vi "Real-Time LED-Core_Process.vi"(0 "FTW Actor Instance Configuration":string="{\n  \"Identity\": \"RT LED\",\n  \"InboxAddress\": \"inproc://rt-led\",\n  \"LoggerAddress\": \"\"\n}", 11 "ErrorIn":errorcluster) -> (15 "Error":errorcluster)   [LabVIEW 2015, in "Real-Time LED-Core.lvclass"]
uses:
  Real-Time LED-Core.lvclass
  Real-Time LED-Core.lvclass/Real-Time LED-Core.ctl
  source/actor/Instance/FTW-ActorInstance.lvclass/FTW-ActorInstance.ctl
  source/actor/JobSequencer/FTW-SEQ-Current.vi
  source/actor/Instance/FTW-ActorInstance.lvclass
  source/actor/Message/Request/FTW-Message-IncomingRequest.lvclass
  <vilib>/NI_Real-Time Target Support.lvlib
panel:
  out "LED":bool
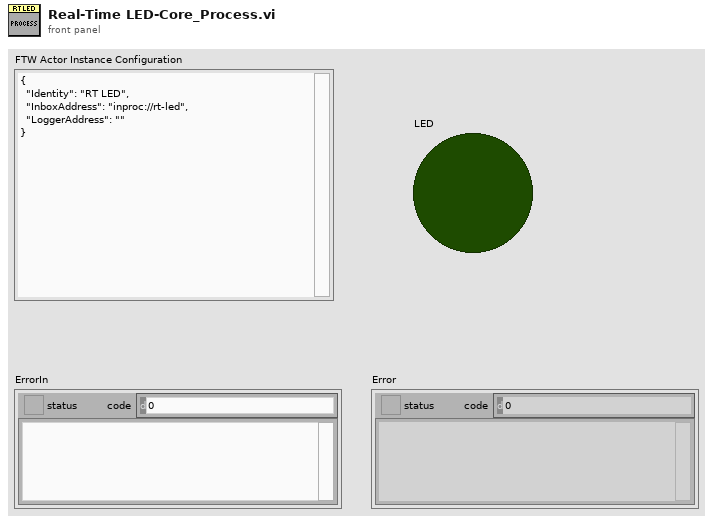
[diagram p1: front panel]
types:
  T1 = cluster{"Incoming Requests":refnum<event-registration>, "Local Messages":refnum<event-registration>, "Subscriber Registration":refnum<event-registration>}
  T2 = cluster{"Period":i32, "Sequence":bool[], "Color":i32}
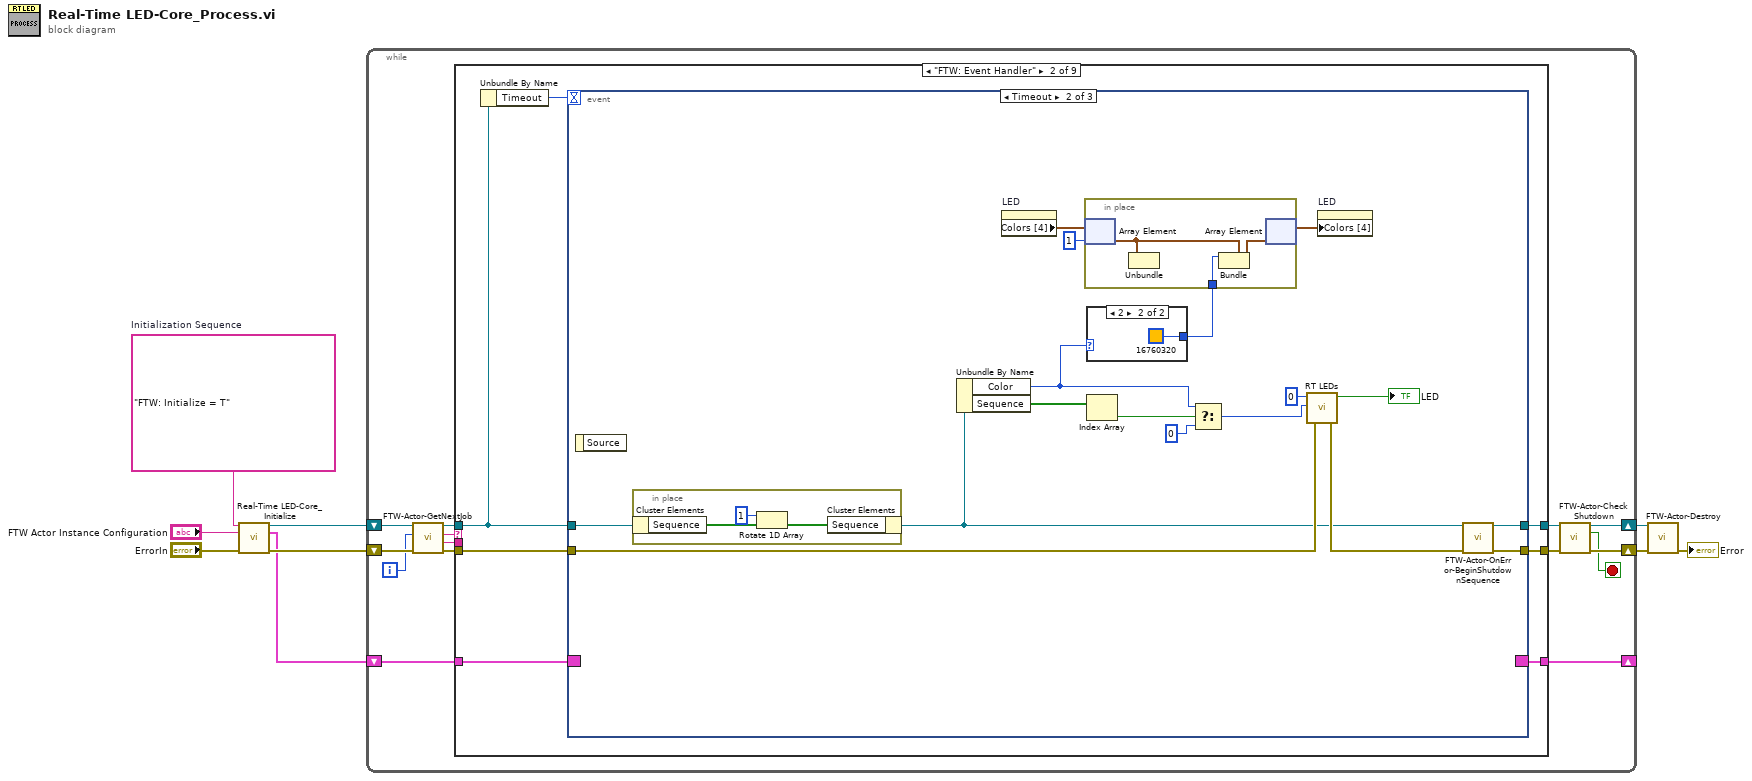
[diagram p0: block diagram]
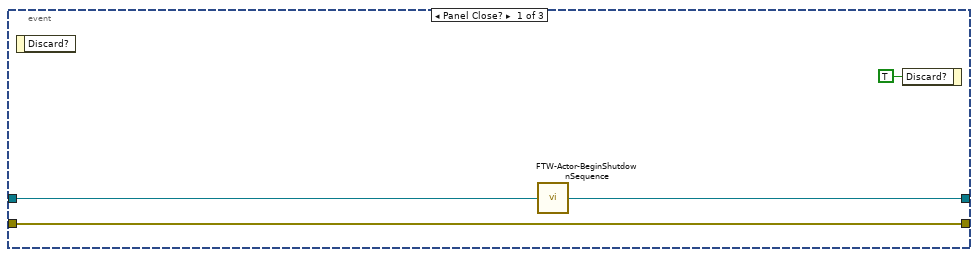
[diagram p3: hidden frame]
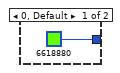
[diagram p4: hidden frame]
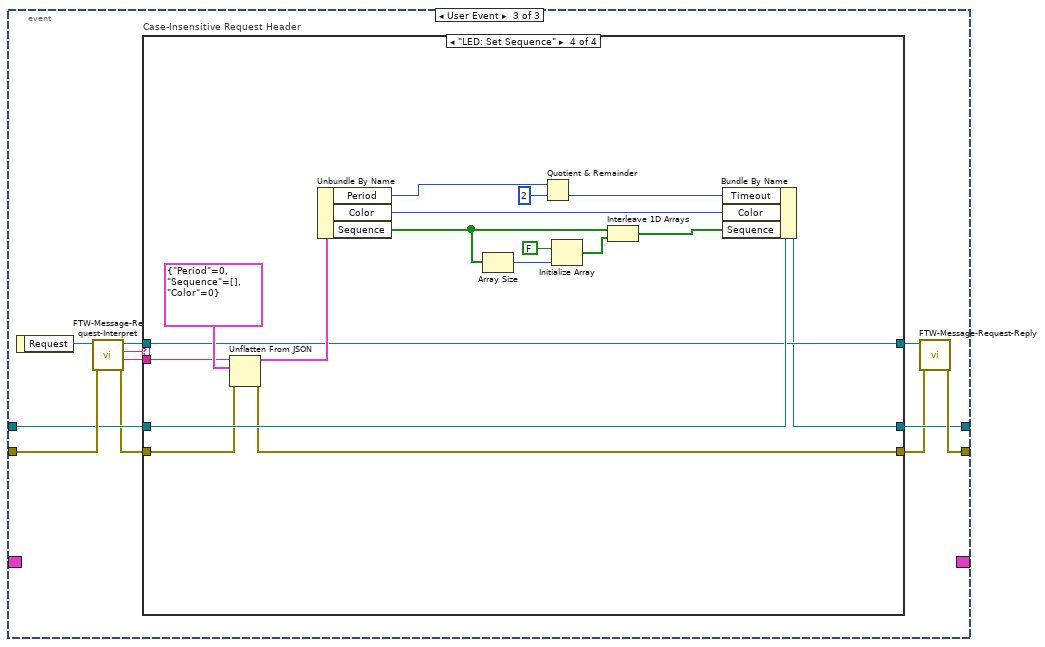
[diagram p5: hidden frame]
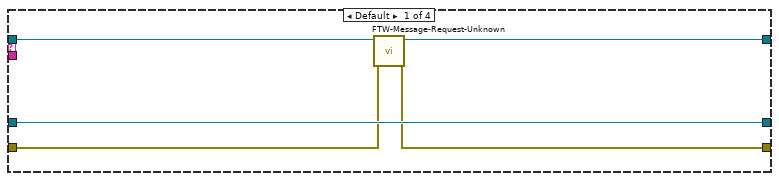
[diagram p6: hidden frame]
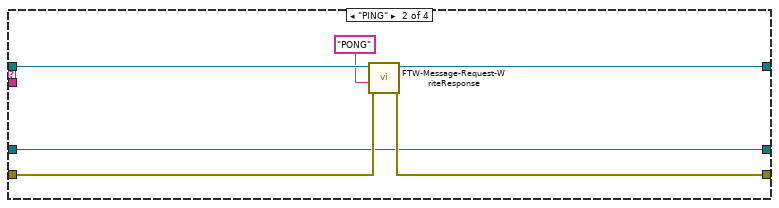
[diagram p7: hidden frame]
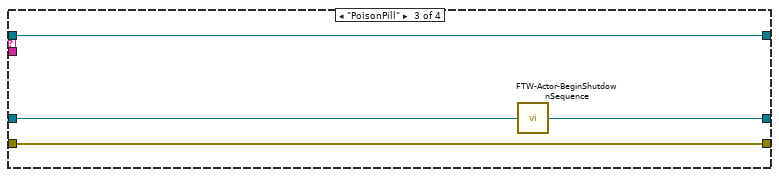
[diagram p8: hidden frame]
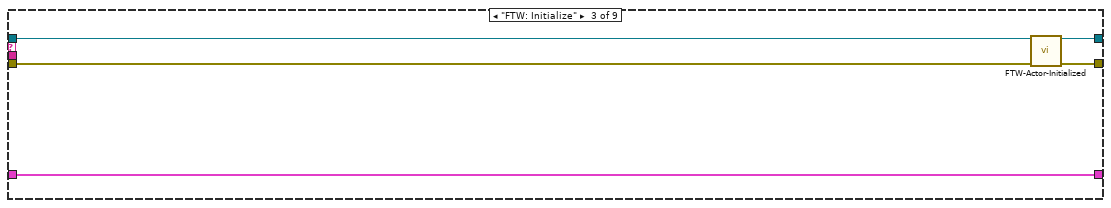
[diagram p9: hidden frame]
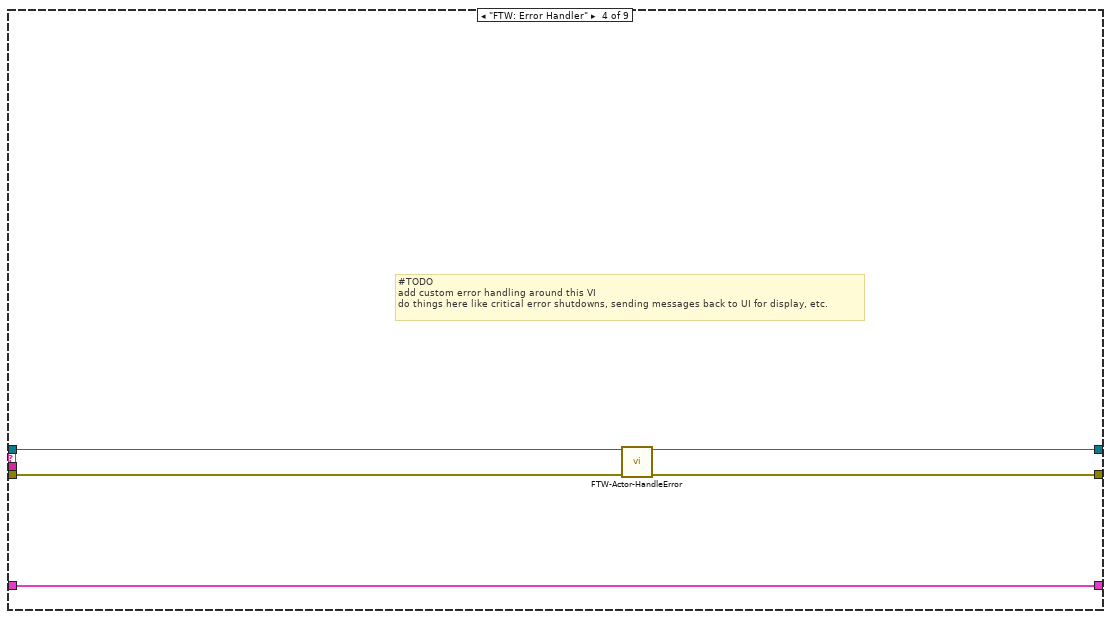
[diagram p10: hidden frame]
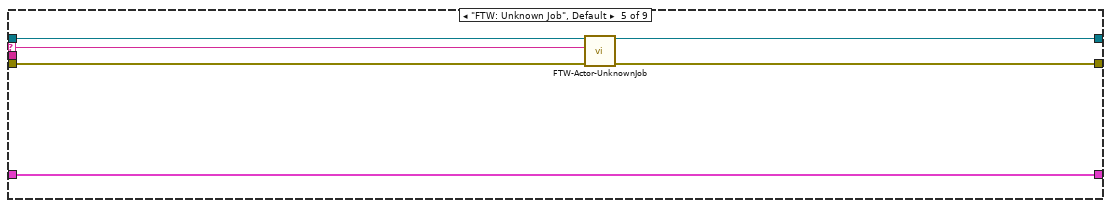
[diagram p11: hidden frame]
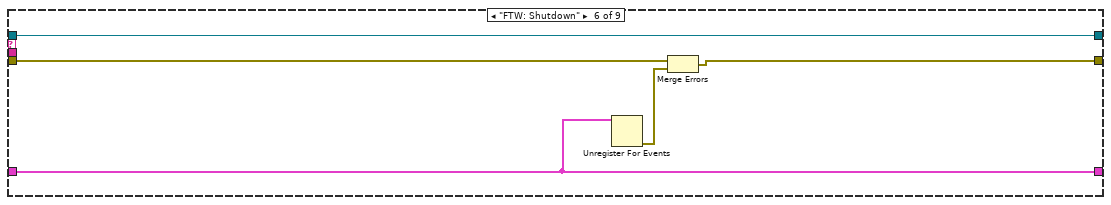
[diagram p12: hidden frame]
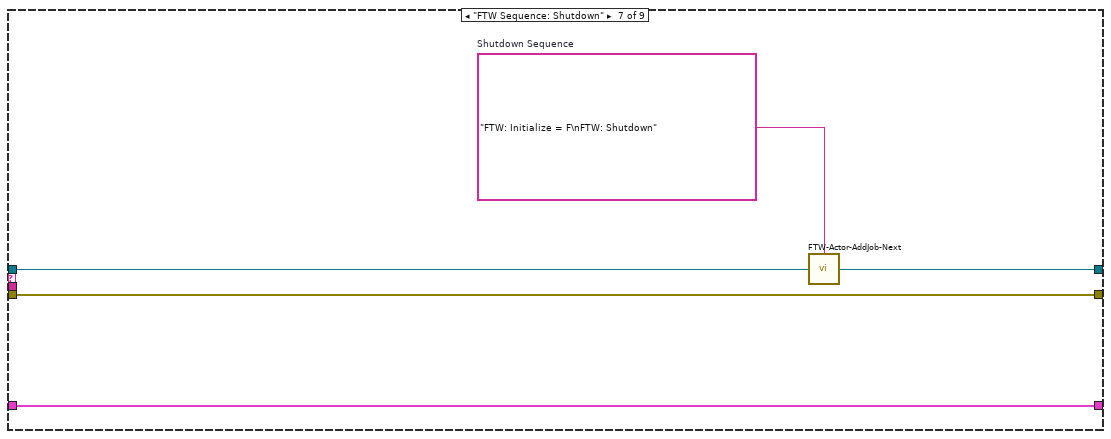
[diagram p13: hidden frame]
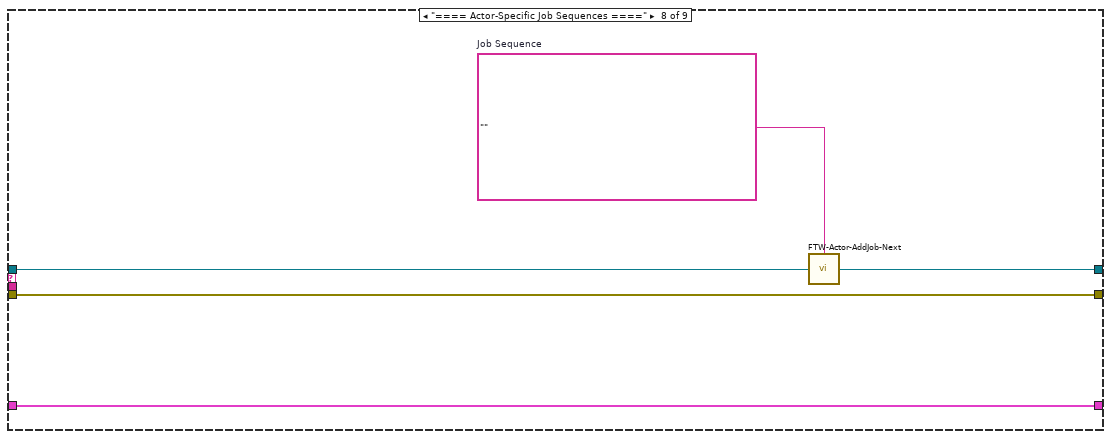
[diagram p14: hidden frame]
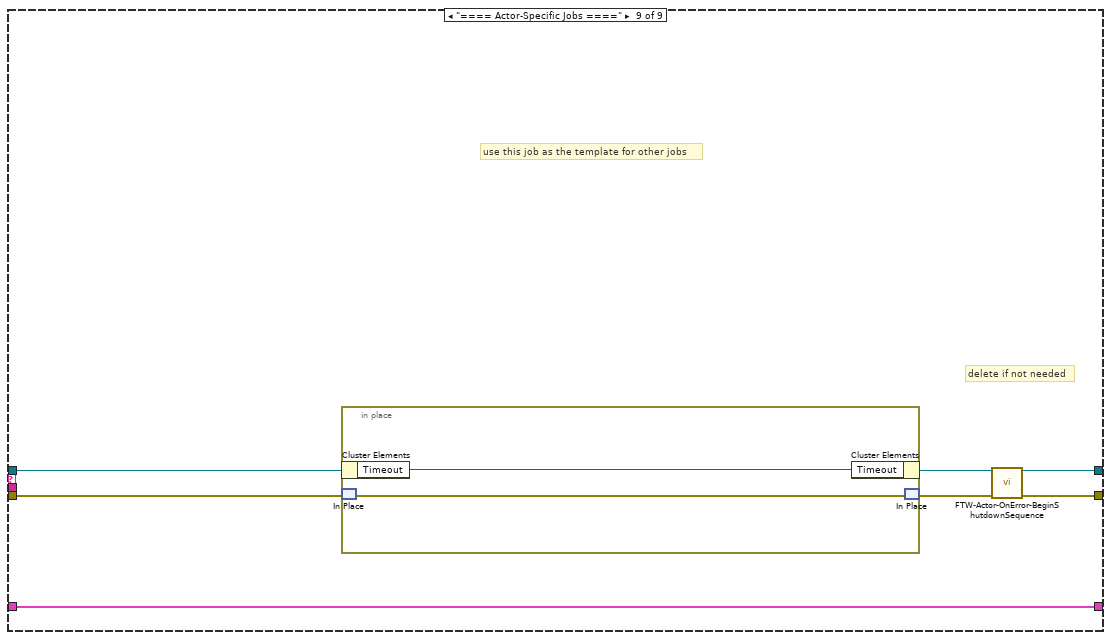
[diagram p15: hidden frame]
diagram:
  w5 = "FTW: Initialize = T"  # Initialization Sequence
  n1 = call "Real-Time LED-Core_Initialize.vi"("Initialization Sequence"=w5, "FTW Actor Instance Configuration"="FTW Actor Instance Configuration", "error in (no error)"="ErrorIn") -> ("Actor Template-Core out"=w1:refnum<class "Real-Time LED-Core.lvclass">, "Event Refnums"=w2:T1, "error out"=w6:errorcluster)  [unwired: 10 in]
  n2 = while {
    shift-right: [w13] -> w8
    shift-left: w6 -> [w20]
    shift-right: [w10] -> _
    shift-left: w2 -> [w23]
    shift-right: [w15] -> w9
    shift-left: w1 -> [w22]
    i -> [w11]
    stop <- w12 stop-if-true
    n3 = call "FTW-Actor-GetNextJob.vi"("error in"=w20, "Jobs Performed"=w11, "FTW Actor Instance"=w22) -> ("error out"=w19:errorcluster, "Job Data"=w17:string, "Job Name"=w18:string, "FTW Actor Instance out"=w21:refnum<class "Real-Time LED-Core.lvclass">)  [unwired: 5 in]
    n4 = case shown="\"FTW: Event Handler\"" w18 {
      selector: w18 -> [_ _ _ _ w116 _ _ _ _]
      tunnel: [w25 w33 w107 w111 w119 w125 w130 w135 w139] -> w14
      tunnel: w19 -> [w25 w32 w109 w113 w120 w126 w130 w135 w142]
      tunnel: w23 -> [w26 w29 w110 w115 w121 w123 w131 w136 w143]
      tunnel: [w26 w31 w110 w115 w121 w123 w131 w136 w143] -> w10
      tunnel: w17 -> [_ _ _ _ _ _ _ _ _]
      tunnel: [w24 w30 w108 w112 w117 w122 w128 w133 w137] -> w16
      tunnel: w21 -> [w24 w28 w106 w114 w118 w122 w129 w134 w140]
      frame "==== Featherweight Framework Jobs ====" {
      }
      frame "FTW: Event Handler" {
        n5 = Unbundle By Name(w28) -> ("Timeout"=w27:i32)
        n6 = event shown="[1] Timeout" {
          selector: w29 -> [_ _ _]
          dyn-events: [_ _ _] -> w31
          timeout: w27 -> [_ _ _]
          tunnel: [w36 w40 w72] -> w33
          tunnel: w32 -> [w36 w54 w71]
          tunnel: [w34 w39 w66] -> w30
          tunnel: w28 -> [w35 w50 w70]
          event Panel Close? {
            n7 = event-data() -> ()  [unwired: 1 in, 1 out]
            n8 = call "FTW-Actor-BeginShutdownSequence.vi"("FTW Actor Instance"=w35) -> ("FTW Actor Instance out"=w34:refnum<class "Real-Time LED-Core.lvclass">)  [unwired: 3 in]
            n9 = event-data("Discard?"=TRUE) -> ()  [unwired: 1 in, 1 out]
          }
          event Timeout {
            n10 = event-data() -> ()  [unwired: 1 in, 1 out]
            n11 = in-place {
              n12 = in-place-cluster #1(w50) -> ("Sequence"=w62:bool[])
              n13 = Rotate 1D Array(1:w62, 2:1 ("n")) -> (0:w61:bool[])
              n14 = in-place-cluster #1("Sequence"=w61) -> (w38:refnum<class "Real-Time LED-Core.lvclass">)
            }
            n15 = Unbundle By Name(w38) -> ("Color"=w43:i32, "Sequence"=w49:bool[])
            n16 = property on="LED" class="Bool (strict)"() -> ("Colors [4]"=w46:cluster{u32, u32}[])  [unwired: 2 in, 2 out]
            n17 = case shown="2" w43 {
              tunnel: [u32 6618880 u32 16760320] -> w42
              frame 0, Default {
              }
              frame 2 {
              }
            }
            n18 = in-place {
              in-place-border: w42 -> [w57]
              n19 = in-place-array #2(w46, 1) -> (w59:cluster{u32, u32})
              n20 = Unbundle(w59) -> ()  [unwired: 2 out]
              n21 = Bundle(cluster=w59, w57) -> (w58:cluster{u32, u32})  [unwired: 1 in]
              n22 = in-place-array #2(w58) -> (w44:cluster{u32, u32}[])  [unwired: 1 out]
            }
            n23 = Index Array(array=w49) -> (element=w48:bool)  [unwired: 1 in]
            n24 = Select(t=w43, s=w48, f=0) -> (s? t:f=w52:i32)
            n25 = call <vilib>:"RT LEDs.vi"("error in (no error)"=w54, "State"=w52, "LED Num"=0) -> ("error out"=w53:errorcluster, "Led State"=→"LED":bool)  [unwired: 3 in]
            n26 = property on="LED" class="Bool (strict)"("Colors [4]"=w44) -> ()  [unwired: 2 in, 2 out]
            n27 = call-dynamic "FTW-Actor-OnError-BeginShutdownSequence.vi"("FTW Actor Instance"=w38, "error in"=w53) -> ("FTW Actor Instance out"=w39:refnum<class "Real-Time LED-Core.lvclass">, "error out"=w40:errorcluster)  [unwired: 12 in]
          }
          event User Event {
            n28 = event-data() -> ("Request"=w73:refnum<class "FTW-Message-IncomingRequest.lvclass">)  [unwired: 1 in]
            n29 = call "FTW-Message-Request-Interpret.vi"("error in"=w71, "FTW Incoming Request"=w73) -> ("error out"=w69:errorcluster, "Request Body"=w63:string, "Request Header"=w67:string, "FTW Incoming Request out"=w68:refnum<class "FTW-Message-IncomingRequest.lvclass">)  [unwired: 6 in]
            n30 = case "Case-Insensitive Request Header" shown="\"LED: Set Sequence\"" w67 {
              tunnel: [w76 w82 w87 w99] -> w65
              tunnel: w69 -> [w77 w83 w87 w102]
              tunnel: [w78 w81 w88 w98] -> w66
              tunnel: w70 -> [w78 w81 w86 w105]
              tunnel: w68 -> [w75 w84 w85 w100]
              tunnel: [w74 w80 w85 w100] -> w64
              tunnel: w63 -> [_ _ _ w101]
              frame Default {
                n31 = call "FTW-Message-Request-Unknown.vi"("error in"=w77, "FTW Incoming Request"=w75) -> ("error out"=w76:errorcluster, "FTW Incoming Request Out"=w74:refnum<class "FTW-Message-IncomingRequest.lvclass">)  [unwired: 8 in]
              }
              frame "PING" {
                n32 = call "FTW-Message-Request-WriteResponse.vi"("error in"=w83, "Response Body"="PONG" ("Response Header"), "FTW Incoming Request"=w84) -> ("error out"=w82:errorcluster, "FTW Incoming Request out"=w80:refnum<class "FTW-Message-IncomingRequest.lvclass">)  [unwired: 7 in]
              }
              frame "PoisonPill" {
                n33 = call "FTW-Actor-BeginShutdownSequence.vi"("FTW Actor Instance"=w86) -> ("FTW Actor Instance out"=w88:refnum<class "Real-Time LED-Core.lvclass">)  [unwired: 3 in]
              }
              frame "LED: Set Sequence" {
                n34 = Unflatten From JSON(JSON string=w101, type and defaults=T2 {"Period"=0, "Sequence"=[], "Color"=0}, error in (no error)=w102) -> (value=w103:T2, error out=w99:errorcluster)  [unwired: 4 in]
                n35 = Unbundle By Name(w103) -> ("Period"=w91:i32, "Color"=w92:i32, "Sequence"=w95:bool[])
                n36 = Array Size(array=w95) -> (size(s)=w97:i32)
                n37 = Quotient & Remainder(x=w91, y=2) -> (floor(x/y)=w90:i32)  [unwired: 1 out]
                n38 = Initialize Array(FALSE, w97) -> (w94:bool[])
                n39 = Interleave 1D Arrays(w95, w94) -> (w93:bool[])
                n40 = Bundle By Name(cluster=w105, "Timeout"=w90, "Color"=w92, "Sequence"=w93) -> (w98:refnum<class "Real-Time LED-Core.lvclass">)
              }
            }
            n41 = call "FTW-Message-Request-Reply.vi"("FTW: Reply Error"=w65, "FTW Incoming Request"=w64) -> ("error out"=w72:errorcluster)  [unwired: 8 in, 1 out]
          }
        }
      }
      frame "FTW: Initialize" {
        n42 = call-dynamic "FTW-Actor-Initialized.vi"("FTW Actor Instance"=w106, "error in"=w109) -> ("FTW Actor Instance out"=w108:refnum<class "Real-Time LED-Core.lvclass">, "error out"=w107:errorcluster)  [unwired: 12 in]
      }
      frame "FTW: Error Handler" {
        # "#TODO\nadd custom error handling around this VI\ndo things here like critical error shutdowns, sending messages back to UI for display, etc."
        n43 = call-dynamic "FTW-Actor-HandleError.vi"("FTW Actor Instance"=w114, "error in"=w113) -> ("FTW Actor Instance out"=w112:refnum<class "Real-Time LED-Core.lvclass">, "error out"=w111:errorcluster)  [unwired: 10 in, 2 out]
      }
      frame "FTW: Unknown Job", Default {
        n44 = call-dynamic "FTW-Actor-UnknownJob.vi"("FTW Actor Instance"=w118, "Unknown Job"=w116, "error in"=w120) -> ("FTW Actor Instance out"=w117:refnum<class "Real-Time LED-Core.lvclass">, "error out"=w119:errorcluster)  [unwired: 11 in]
      }
      frame "FTW: Shutdown" {
        n45 = Unregister For Events(event registration refnum=w123) -> (error out=w124:errorcluster)  [unwired: 1 in]
        n46 = Merge Errors(w126, w124) -> (w125:errorcluster)
      }
      frame "FTW Sequence: Shutdown" {
        w127 = "FTW: Initialize = F\nFTW: Shutdown"  # Shutdown Sequence
        n47 = call "FTW-Actor-AddJob-Next.vi"("Add Next in Job Queue"=w127, "FTW Actor Instance"=w129) -> ("FTW Actor Instance out"=w128:refnum<class "Real-Time LED-Core.lvclass">)  [unwired: 2 in]
      }
      frame "==== Actor-Specific Job Sequences ====" {
        w132 = ""  # Job Sequence
        n48 = call "FTW-Actor-AddJob-Next.vi"("Add Next in Job Queue"=w132, "FTW Actor Instance"=w134) -> ("FTW Actor Instance out"=w133:refnum<class "Real-Time LED-Core.lvclass">)  [unwired: 2 in]
      }
      frame "==== Actor-Specific Jobs ====" {
        # "delete if not needed"
        # "use this job as the template for other jobs"
        n49 = in-place {
          n50 = in-place-cluster #3(w140) -> ("Timeout"=w144:i32)
          n51 = in-place-match #4(w142) -> (w145:errorcluster)
          n52 = in-place-cluster #3("Timeout"=w144) -> (w138:refnum<class "Real-Time LED-Core.lvclass">)
          n53 = in-place-match #4(w145) -> (w141:errorcluster)
        }
        n54 = call-dynamic "FTW-Actor-OnError-BeginShutdownSequence.vi"("FTW Actor Instance"=w138, "error in"=w141) -> ("FTW Actor Instance out"=w137:refnum<class "Real-Time LED-Core.lvclass">, "error out"=w139:errorcluster)  [unwired: 12 in]
      }
    }
    n55 = call "FTW-Actor-CheckShutdown.vi"("FTW Actor Instance"=w16, "error in"=w14) -> ("FTW Actor Instance out"=w15:refnum<class "Real-Time LED-Core.lvclass">, "Shutdown?"=w12:bool, "error out"=w13:errorcluster)  [unwired: 11 in]
  }
  n56 = call-dynamic "FTW-Actor-Destroy.vi"("FTW Actor Instance"=w9, "error in"=w8) -> ("error out"=→"Error":errorcluster)  [unwired: 13 in]
